vi "Beampointing get set motor position.vi"(7 "Active CCD":i32, 8 "error in (no error)":errorcluster, 9 "Set position":dbl, 10 "get or set":enum16{"get", "set"}(ring)=enum."set", 11 "dev variable alias Motors X":string[][](array[string])) -> (0 "error out":errorcluster, 3 "Actual Position":dbl)   [LabVIEW 2020]
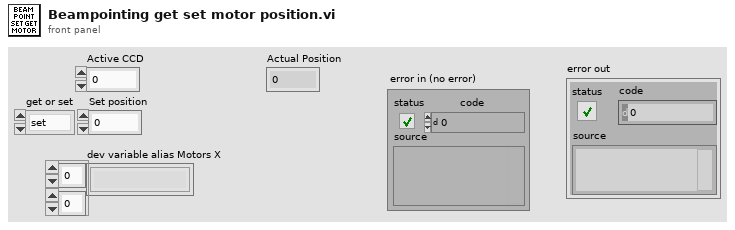
[diagram p1: front panel]
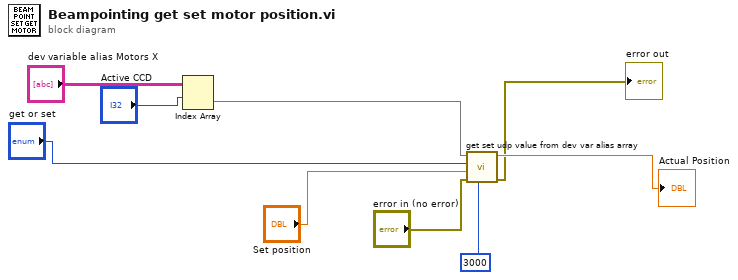
[diagram p0: block diagram]
diagram:
  n1 = Index Array(array="dev variable alias Motors X", index (row)="Active CCD") -> (element=w9:string[])  [unwired: 1 in]
  n2 = call "get set udp value from dev var alias array.vi"("slow timeout ms (3000)"=3000, "error in (no error)"="error in (no error)", "Set position"="Set position", "get or set"="get or set", "dev variable alias Motors X"=w9) -> ("error out"=→"error out":errorcluster, "Numeric"=→"Actual Position":dbl)  [unwired: 5 in]
